vi "Class.Flatten.vi"(8 "error in (no error)":errorcluster, 11 "Data Access API in":refnum<class "Data Access API.lvclass">) -> (0 "error out":errorcluster, 2 "Flattened Class":string, 3 "Data Access API out":refnum<class "Data Access API.lvclass">)   [LabVIEW 2015, in "Data Access API.lvlib" / "Data Access API.lvclass"]
uses:
  Data Access API.lvclass
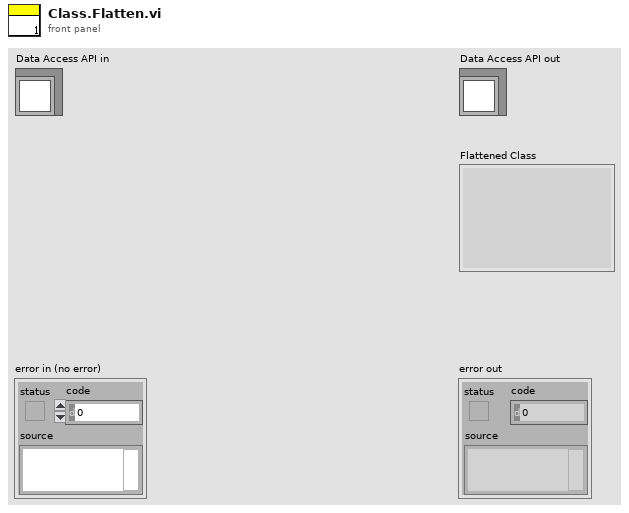
[diagram p1: front panel]
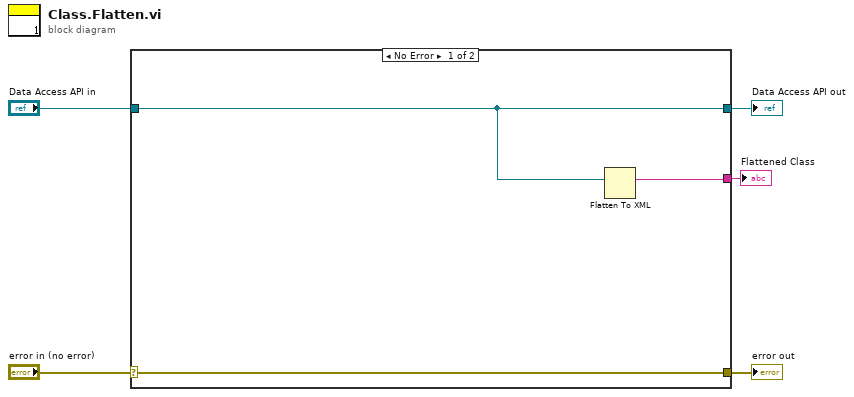
[diagram p0: block diagram]
diagram:
  n1 = case shown="No Error" "error in (no error)" {
    selector: "error in (no error)" -> [w8 w10]
    tunnel: [w8 w10] -> w4
    tunnel: [w7 w9] -> w2
    tunnel: "Data Access API in" -> [w7 w9]
    tunnel: [w6 _] -> w1
    frame No Error {
      n2 = Flatten To XML(anything=w7) -> (xml string=w6:string)
    }
    frame Error {
    }
  }
  "error out" <- w4
  "Data Access API out" <- w2
  "Flattened Class" <- w1
